vi "Save-exec-script.vi"(8 "error in":errorcluster, 10 "Script array":T1[](array[typedef]), 11 "file (use dialog)":path=path "C:/Projects/Alpha Redux/Script.csv") -> (0 "error out":errorcluster, 3 "Script string":string)   [LabVIEW 2021]
uses:
  Controls/Command_Enum.ctl
  Controls/Command_cluster.ctl
  <vilib>/Utility/error.llb/whitespace.ctl
panel:
  in  "Commands":T2=enum."Y Home"
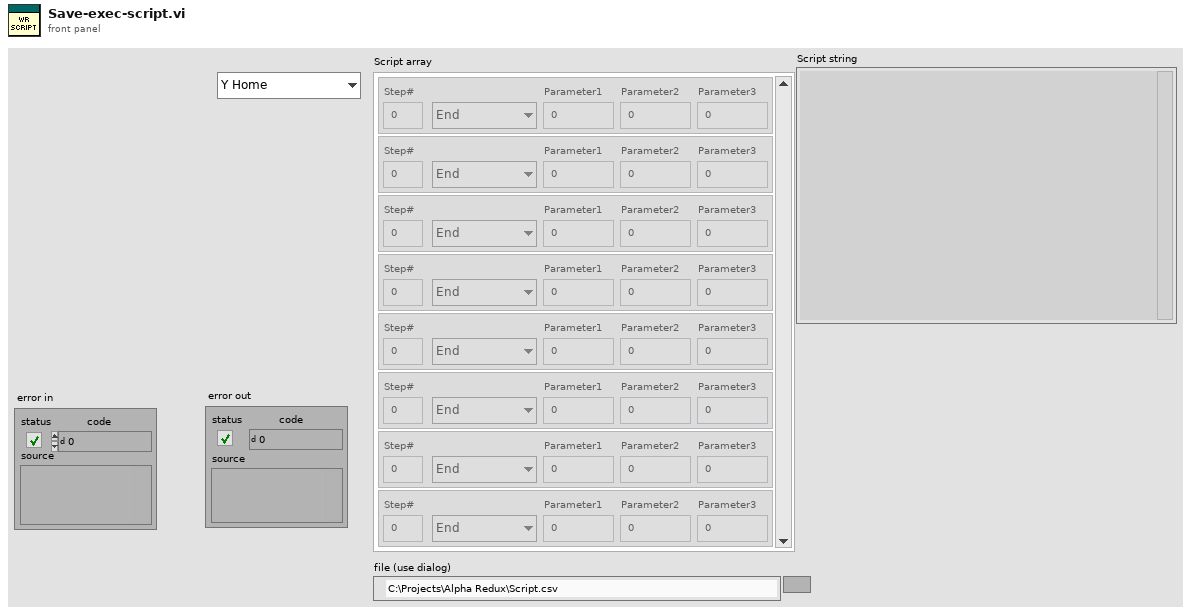
[diagram p1: front panel]
types:
  T1 = typedef "Command_cluster.ctl" = cluster{"Step#":dbl, "Commands":T2, "Parameter1":dbl, "Parameter2":dbl, "Parameter3":dbl}
  T2 = typedef "Command_Enum.ctl" = enum16{"End", "Home All", "X Home", "Y Home", "X Move Rel", "X Move Abs", "Y Move Rel", "Y Move Abs", "Wait", "Repeat"}
  T3 = typedef "whitespace.ctl" = u16
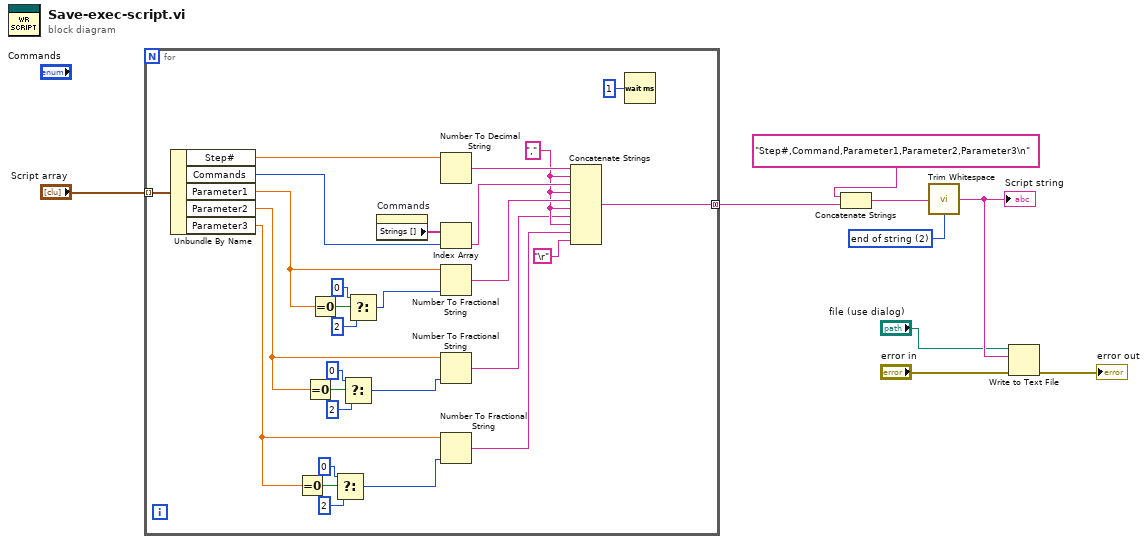
[diagram p0: block diagram]
diagram:
  w5 = T3 2 items=["both", "start of string", "end of string"] ("location (both)")
  n1 = for {
    tunnel: "Script array" -> [w37] mode=indexing
    tunnel: [w27] -> w7 mode=concatenating
    w29 = ","
    n2 = Unbundle By Name(w37) -> ("Step#"=w36:dbl, "Commands"=w35:T2, "Parameter1"=w25:dbl, "Parameter2"=w15:dbl, "Parameter3"=w14:dbl)
    n3 = Equal To 0?(x=w14) -> (x = 0?=w18:bool)
    n4 = Equal To 0?(x=w15) -> (x = 0?=w21:bool)
    n5 = Equal To 0?(x=w25) -> (x = 0?=w24:bool)
    n6 = Select(t=i16 0 ("precision (6)"), s=w18, f=i16 2 ("precision (6)")) -> (s? t:f=w10:i16)
    n7 = Select(t=i16 0 ("precision (6)"), s=w21, f=i16 2 ("precision (6)")) -> (s? t:f=w11:i16)
    n8 = Select(t=i16 0 ("precision (6)"), s=w24, f=i16 2 ("precision (6)")) -> (s? t:f=w13:i16)
    n9 = property on="Commands" class="Enum (strict)"() -> ("Strings []"=w34:string[])  [unwired: 2 in, 2 out]
    n10 = Number To Decimal String(number=w36) -> (decimal integer string=w33:string)  [unwired: 1 in]
    n11 = Index Array(array=w34, index=w35) -> (element=w32:string)
    n12 = Number To Fractional String(number=w25, precision (6)=w13) -> (F-format string=w31:string)  [unwired: 2 in]
    n13 = Number To Fractional String(number=w15, precision (6)=w11) -> (F-format string=w12:string)  [unwired: 2 in]
    n14 = Number To Fractional String(number=w14, precision (6)=w10) -> (F-format string=w30:string)  [unwired: 2 in]
    n15 = Concatenate Strings(w33, w29, w32, w29, w31, w29, w12, w29, w30, "\r") -> (w27:string)
    n16 = Wait (ms)(milliseconds to wait=u32 1) -> ()  [unwired: 1 out]
  }
  n17 = Concatenate Strings("Step#,Command,Parameter1,Parameter2,Parameter3\n", w7) -> (w6:string)
  n18 = call <vilib>:"Trim Whitespace.vi"("string"=w6, "location (both)"=w5) -> ("trimmed string"=w2:string)
  "Script string" <- w2
  n19 = Write to Text File(file (use dialog)="file (use dialog)", text=w2, error in="error in") -> (error out=→"error out":errorcluster)  [unwired: 1 in, 2 out]
